vi "POP_Init Controls.vi"(8 "Error In":errorcluster caption="错误输入（无错误）", 9 "Font Size":u32, 10 "TontName":string="Tahoma", 11 "Popup Cluster Ref":refnum<vi>) -> (0 "Error Out":errorcluster caption="错误输入（无错误）", 2 "Offsets":cluster{"Left":i32, "Top":i32}[](array[cluster]), 3 "Popup Cluster Ref Out":refnum<vi>)   [LabVIEW 2016]
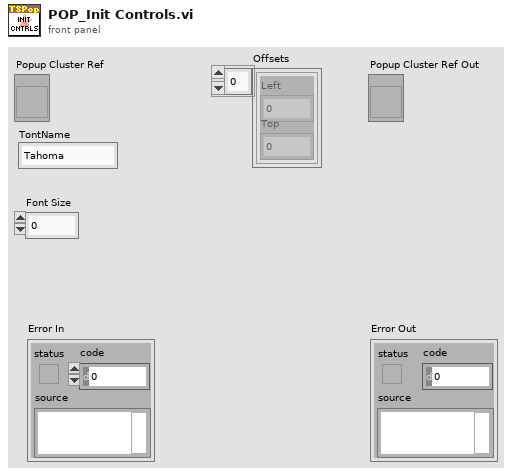
[diagram p1: front panel]
types:
  T1 = typedef "LVPositionTypeDef.ctl" = cluster{"Left":i32, "Top":i32}
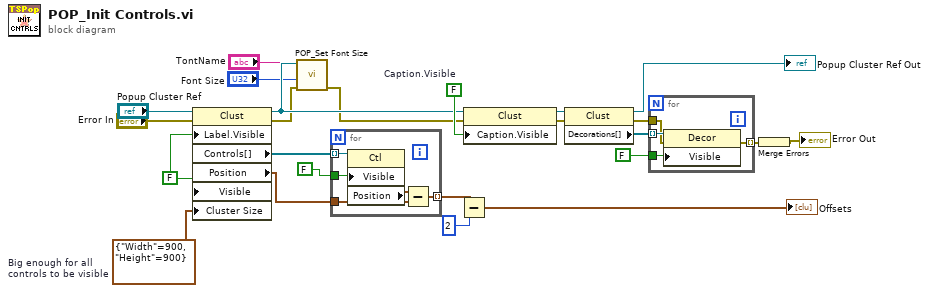
[diagram p0: block diagram]
diagram:
  w12 = FALSE  # Caption.Visible
  w20 = cluster{"Width":u32, "Height":u32} {"Width"=900, "Height"=900}  # Big enough for all controls to be visible
  w21 = FALSE ("Wait until done")
  n1 = property class="Clust"(reference="Popup Cluster Ref", error in="Error In", "Label.Visible"=w21, "Visible"=w21, "Cluster Size"=w20) -> (reference out=w10:refnum<vi>, error out=w8:errorcluster, "Controls[]"=w11:refnum<vi>[], "Position"=w15:T1)
  n2 = call "POP_Set Font Size.vi"("error in (no error)"=w8, "Font Size"="Font Size", "TontName"="TontName", "Popup Cluster Ref"=w10) -> ("error out"=w7:errorcluster)  [unwired: 6 in, 1 out]
  n3 = for {
    tunnel: w11 -> [w29] mode=indexing
    tunnel: w15 -> [w27]
    tunnel: [w26] -> w22 mode=indexing
    tunnel: FALSE ("Wait until done") -> [w25]
    n4 = property class="Ctl"(reference=w29, "Visible"=w25) -> ("Position"=w28:T1)  [unwired: 1 in, 2 out]
    n5 = Subtract(x=w28, y=w27) -> (x-y=w26:T1)
  }
  n6 = Subtract(x=w22, y=2) -> (x-y=→"Offsets":T1[])
  n7 = property class="Clust"(reference=w10, error in=w7, "Caption.Visible"=w12) -> (reference out=w13:refnum<vi>, error out=w6:errorcluster)
  n8 = property class="Clust"(reference=w13, error in=w6) -> (reference out=→"Popup Cluster Ref Out":refnum<vi>, error out=w4:errorcluster, "Decorations[]"=w18:refnum<vi>[])
  n9 = for {
    tunnel: w18 -> [w33] mode=indexing
    tunnel: FALSE ("Visible") -> [w32]
    tunnel: w4 -> [w31]
    tunnel: [w30] -> w3 mode=indexing
    n10 = property class="Decor"(reference=w33, error in=w31, "Visible"=w32) -> (error out=w30:errorcluster)  [unwired: 1 out]
  }
  n11 = Merge Errors(w3) -> (→"Error Out":errorcluster)
